vi "SelectMenu5.vi"(0 "XRef":T10, 1 "Tag":T5, 2 "Point":T8, 3 "Menu Type":T7, 4 "State In":T1) -> (14 "Reply":T4, 15 "Handled?":T6, 16 "Multi Object Popup Options":T3, 17 "Fatal Error Out":T2, 18 "State Out":T1)   [LabVIEW 2015, in "Get Object Parameters.xnode"]
uses:
  Get Object Parameters.xnode
  <vilib>/XNodeSupport/XNodeXNodeRef.ctl
  <vilib>/XNodeSupport/XNodeString.ctl
  <vilib>/XNodeSupport/XNodePoint.ctl
  <vilib>/XNodeSupport/XNodeInt.ctl
  <vilib>/XNodeSupport/XNodeMenuType.ctl
  State.ctl
  <vilib>/XNodeSupport/XNodeStringArray.ctl
  <vilib>/XNodeSupport/XNodeBool.ctl
  <vilib>/XNodeSupport/XNodeMultiObjectPopupOptions.ctl
  <vilib>/XNodeSupport/XNodeErrorCluster.ctl
  dimensions.vi
  <vilib>/XNodeSupport/NI_XNodeSupport.lvlib
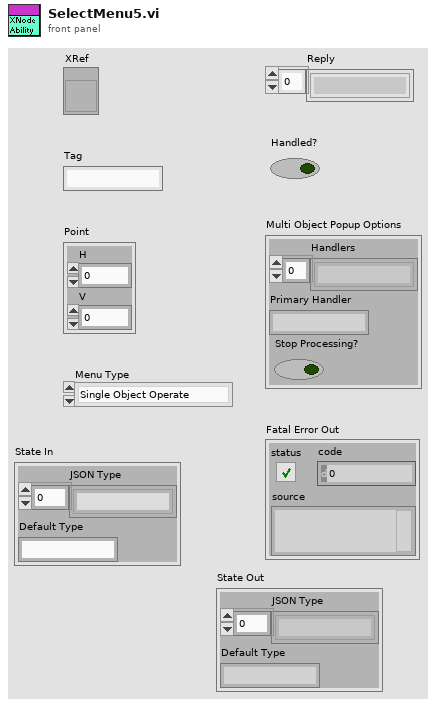
[diagram p1: front panel]
types:
  T1 = typedef "Get Object Parameters.xnode/State.ctl" = cluster{"JSON Type":string[], "Default Type":string}
  T2 = typedef "NI_XNodeSupport.lvlib/XNodeErrorCluster.ctl" = errorcluster
  T3 = typedef "NI_XNodeSupport.lvlib/XNodeMultiObjectPopupOptions.ctl" = cluster{"Handlers":T4, "Primary Handler":T5, "Stop Processing?":T6}
  T4 = typedef "NI_XNodeSupport.lvlib/XNodeStringArray.ctl" = T5[]
  T5 = typedef "NI_XNodeSupport.lvlib/XNodeString.ctl" = string
  T6 = typedef "NI_XNodeSupport.lvlib/XNodeBool.ctl" = bool
  T7 = typedef "NI_XNodeSupport.lvlib/XNodeMenuType.ctl" = enum32{"Single Object Operate", "Single Object Popup", "Multi Object Popup Master", "Multi Object Popup Other"}
  T8 = typedef "NI_XNodeSupport.lvlib/XNodePoint.ctl" = cluster{"H":T9, "V":T9}
  T9 = typedef "NI_XNodeSupport.lvlib/XNodeInt.ctl" = i32
  T10 = typedef "NI_XNodeSupport.lvlib/XNodeXNodeRef.ctl" = refnum<vi>
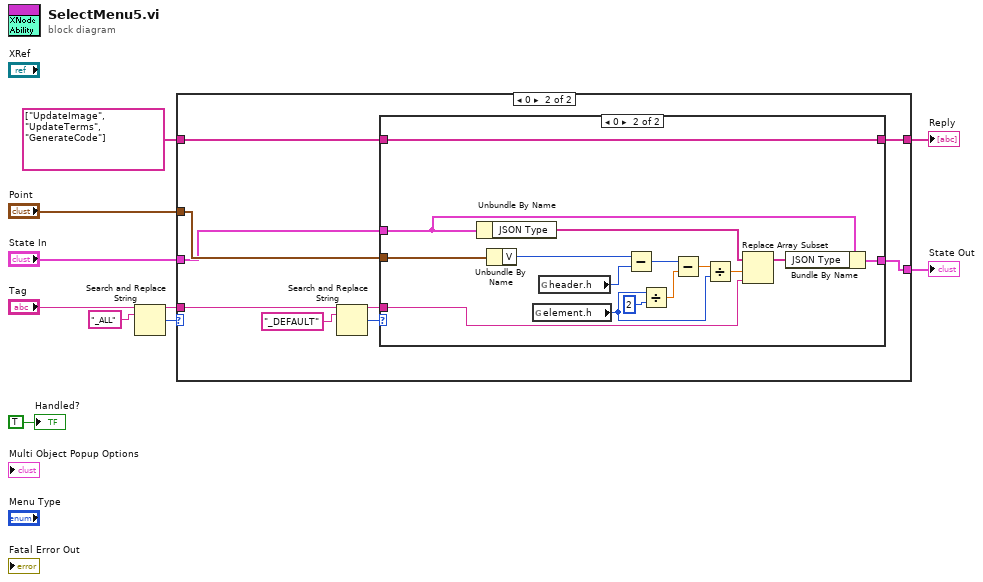
[diagram p0: block diagram]
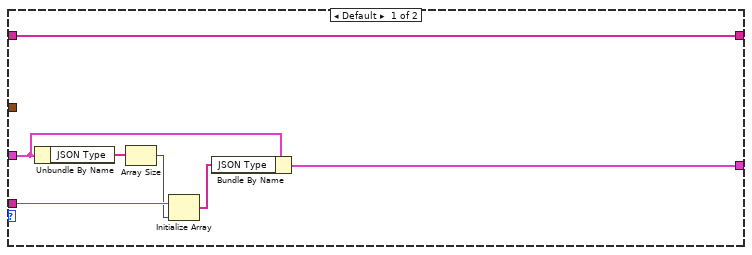
[diagram p2: hidden frame]
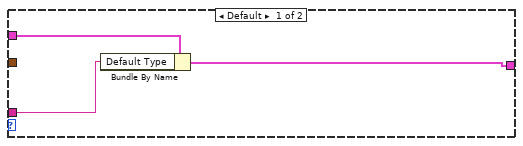
[diagram p3: hidden frame]
diagram:
  n1 = Search and Replace String(input string="Tag", search string="_ALL") -> (result string=w3:string, number of replacements=w4:i32)  [unwired: 6 in, 2 out]
  n2 = case shown="0" w4 {
    tunnel: "Point" -> [_ w26]
    tunnel: "State In" -> [w17 w25]
    tunnel: [w15 w24] -> w7
    tunnel: w3 -> [w14 w22]
    tunnel: T4 ["UpdateImage", "UpdateTerms", "GenerateCode"] ("Reply") -> [w11 w19]
    tunnel: [w11 w18] -> w1
    frame Default {
      n3 = Unbundle By Name(w17) -> ("JSON Type"=w13:string[])
      n4 = Array Size(array=w13) -> (size(s)=w12:i32)
      n5 = Initialize Array(w14, w12) -> (w16:string[])
      n6 = Bundle By Name(cluster=w17, "JSON Type"=w16) -> (w15:T1)
    }
    frame 0 {
      n7 = Search and Replace String(input string=w22, search string="_DEFAULT") -> (result string=w21:string, number of replacements=w20:i32)  [unwired: 6 in, 2 out]
      n8 = case shown="0" w20 {
        tunnel: w26 -> [_ w44]
        tunnel: w25 -> [w29 w41]
        tunnel: [w27 w39] -> w24
        tunnel: w21 -> [w28 w38]
        tunnel: w19 -> [_ w30]
        tunnel: [_ w30] -> w18
        frame Default {
          n9 = Bundle By Name(cluster=w29, "Default Type"=w28) -> (w27:T1)
        }
        frame 0 {
          n10 = Unbundle By Name(w41) -> ("JSON Type"=w42:string[])
          n11 = Unbundle By Name(w44) -> ("V"=w37:T9)
          n12 = global read "dimensions.vi" "element.h"() -> (w34:i16)
          n13 = global read "dimensions.vi" "header.h"() -> (w43:i16)
          n14 = Subtract(x=w37, y=w43) -> (x-y=w35:T9)
          n15 = Divide(x=w34, y=i16 2) -> (x/y=w32:dbl)
          n16 = Subtract(x=w35, y=w32) -> (x-y=w31:dbl)
          n17 = Divide(x=w31, y=w34) -> (x/y=w36:dbl)
          n18 = Replace Array Subset(array=w42, new element=w38, index=w36) -> (w40:string[])
          n19 = Bundle By Name(cluster=w41, "JSON Type"=w40) -> (w39:T1)
        }
      }
    }
  }
  "Reply" <- w1
  "State Out" <- w7
  "Handled?" <- T6 TRUE ("Handled?")
